vi "Rec_CAN_MsgList.vi"(8 "错误输入（无错误）":errorcluster, 9 "AOnlyRx":u8, 10 "AAppChannel输入":i32, 11 "ACANBufferSize":i32) -> (0 "错误输出":errorcluster, 1 "tsapp_receive_can_message":bool, 2 "tsapp_receive_can_messageList":T1[](array[typedef]))   [LabVIEW 2016]
uses:
  SubVIs/MessageInfo.ctl
  SubVIs/SendMsgInfo.ctl
  TSMaster.dll
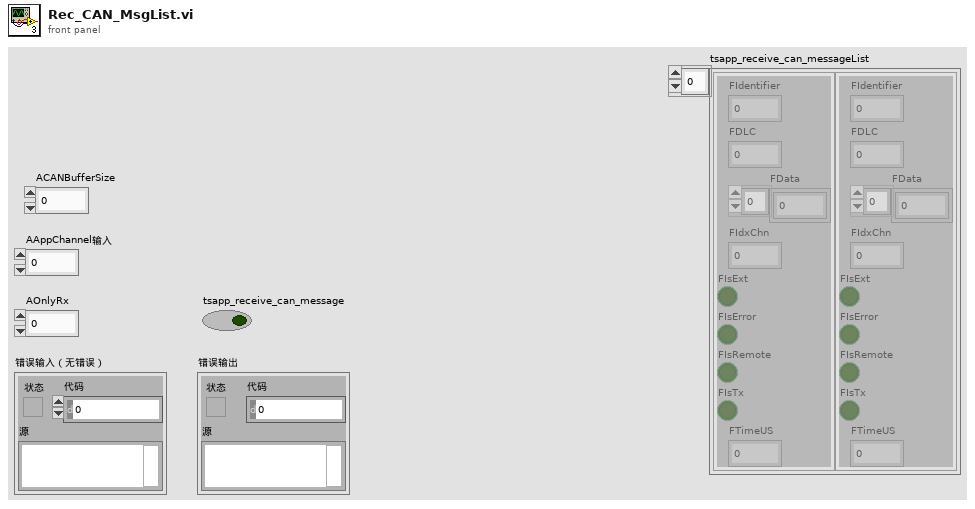
[diagram p1: front panel]
types:
  T1 = typedef "MessageInfo.ctl" = cluster{"FIdentifier":i32, "FDLC":u8, "FData":u8[], "FIdxChn":u8, "FIsExt":bool, "FIsError":bool, "FIsRemote":bool, "FIsTx":bool, "FTimeUS":u64}
  T2 = typedef "SendMsgInfo.ctl" = cluster{"FIdxChn":u8, "FProperties":u8, "FDLC":u8, "FReserved":u8, "FIdentifier":i32, "FTimeUS":u64, "Data0":u8, "Data1":u8, "Data2":u8, "Data3":u8, "Data4":u8, "Data5":u8, "Data6":u8, "Data7":u8}
  T3 = typedef "TCANProperty.ctl" = cluster{"istx":bool, "remoteframe":bool, "extframe":bool, "tbd1":bool, "tbd2":bool, "tbd3":bool, "tbd4":bool, "iserrorframe":bool}
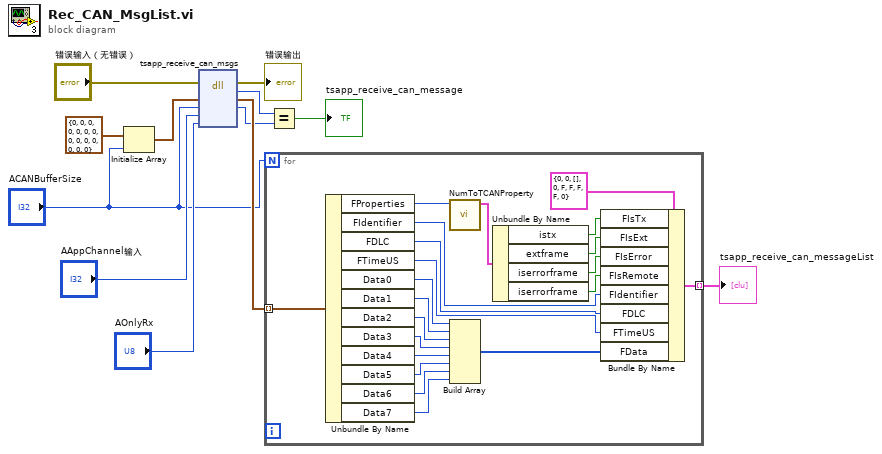
[diagram p0: block diagram]
diagram:
  n1 = Initialize Array(T2 {"FIdxChn"=0, "FProperties"=0, "FDLC"=0, "FReserved"=0, "FIdentifier"=0, "FTimeUS"=0, "Data0"=0, "Data1"=0, "Data2"=0, "Data3"=0, "Data4"=0, "Data5"=0, "Data6"=0, "Data7"=0} ("SendMsgInfo"), "ACANBufferSize") -> (w3:T2[])
  n2 = dll-call lib="C:/Users/Eric/Desktop/LabVIEW/TSMasterAPI/Win32/CANopen_TS_2015/TSMaster.dll" fn="tsapp_receive_can_msgs"(error in="错误输入（无错误）", "ACANBuffers"=w3, "ACANBufferSize"="ACANBufferSize", "AChn"="AAppChannel输入", "ARxTx"="AOnlyRx") -> (error out=→"错误输出":errorcluster, "tsapp_receive_can_msgs"=w6:i32, "ACANBuffers"=w7:T2[], "ACANBufferSize"=w5:i32)  [unwired: 4 in, 1 out]
  n3 = for {
    N: "ACANBufferSize" -> [_]
    tunnel: [w33] -> w1 mode=indexing
    tunnel: w7 -> [w31] mode=indexing
    n4 = Unbundle By Name(w31) -> ("FProperties"=w30:u8, "FIdentifier"=w24:i32, "FDLC"=w23:u8, "FTimeUS"=w22:u64, "Data0"=w21:u8, "Data1"=w20:u8, "Data2"=w19:u8, "Data3"=w18:u8, "Data4"=w17:u8, "Data5"=w16:u8, "Data6"=w15:u8, "Data7"=w14:u8)
    n5 = call "NumToTCANProperty.vi"("TCANPropertyNum"=w30) -> ("TCANProperty"=w29:T3)  [unwired: 10 in]
    n6 = Build Array(w21, w20, w19, w18, w17, w16, w15, w14) -> (w13:u8[])
    n7 = Unbundle By Name(w29) -> ("istx"=w28:bool, "extframe"=w27:bool, "iserrorframe"=w26:bool, "iserrorframe"=w25:bool)
    n8 = Bundle By Name(cluster=T1 {"FIdentifier"=0, "FDLC"=0, "FData"=[], "FIdxChn"=0, "FIsExt"=FALSE, "FIsError"=FALSE, "FIsRemote"=FALSE, "FIsTx"=FALSE, "FTimeUS"=0} ("Receive message"), "FIsTx"=w28, "FIsExt"=w27, "FIsError"=w26, "FIsRemote"=w25, "FIdentifier"=w24, "FDLC"=w23, "FTimeUS"=w22, "FData"=w13) -> (w33:T1)
  }
  "tsapp_receive_can_messageList" <- w1
  n9 = Equal?(x=w6, y=w5) -> (x = y?=→"tsapp_receive_can_message":bool)
